vi "Open HVPS.vi"(8 "error in":errorcluster, 11 "DAQ HVPS in":refnum<class "DAQ HVPS.lvclass">) -> (0 "error out":errorcluster, 3 "DAQ HVPS out":refnum<class "DAQ HVPS.lvclass">)   [LabVIEW 2014, in "DAQ HVPS.lvclass"]
doc: "Use this method to establish connections to the HVPS."
uses:
  Session Based/DAQ/DAQ HVPS.lvclass
  DAQ HVPS.lvclass
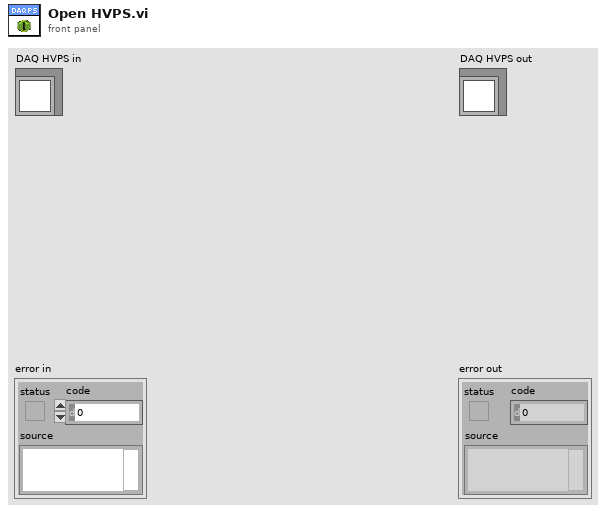
[diagram p1: front panel]
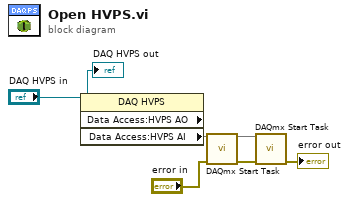
[diagram p0: block diagram]
diagram:
  n1 = property class="DAQ HVPS"(reference="DAQ HVPS in") -> ("Data Access:HVPS AO"=w3, "Data Access:HVPS AI"=w1)  [unwired: 1 in, 2 out]
  n2 = call <vilib>:"DAQmx Start Task.vi"("task/channels in"=w1, "error in"="error in") -> ("error out"=w6:errorcluster)  [unwired: 12 in, 1 out]
  n3 = call <vilib>:"DAQmx Start Task.vi"("task/channels in"=w3, "error in"=w6) -> ("error out"=→"error out":errorcluster)  [unwired: 12 in, 1 out]
  "DAQ HVPS out" <- "DAQ HVPS in"
